vi "读取倍频程数据.vi"(8 "error in (no error)":errorcluster caption="错误输入（无错误）", 10 "写入缓冲区":string, 11 "设备选择":refnum<visa-resource-name>) -> (0 "error out":errorcluster caption="错误输出", 1 "read OCT":string, 2 "read SLM":string, 3 "通道编号输出":u32)   [LabVIEW 2020, in "bas_meas.lvlib"]
uses:
  bas_meas.lvlib
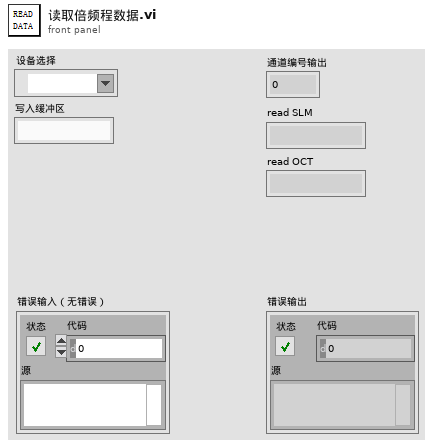
[diagram p1: front panel]
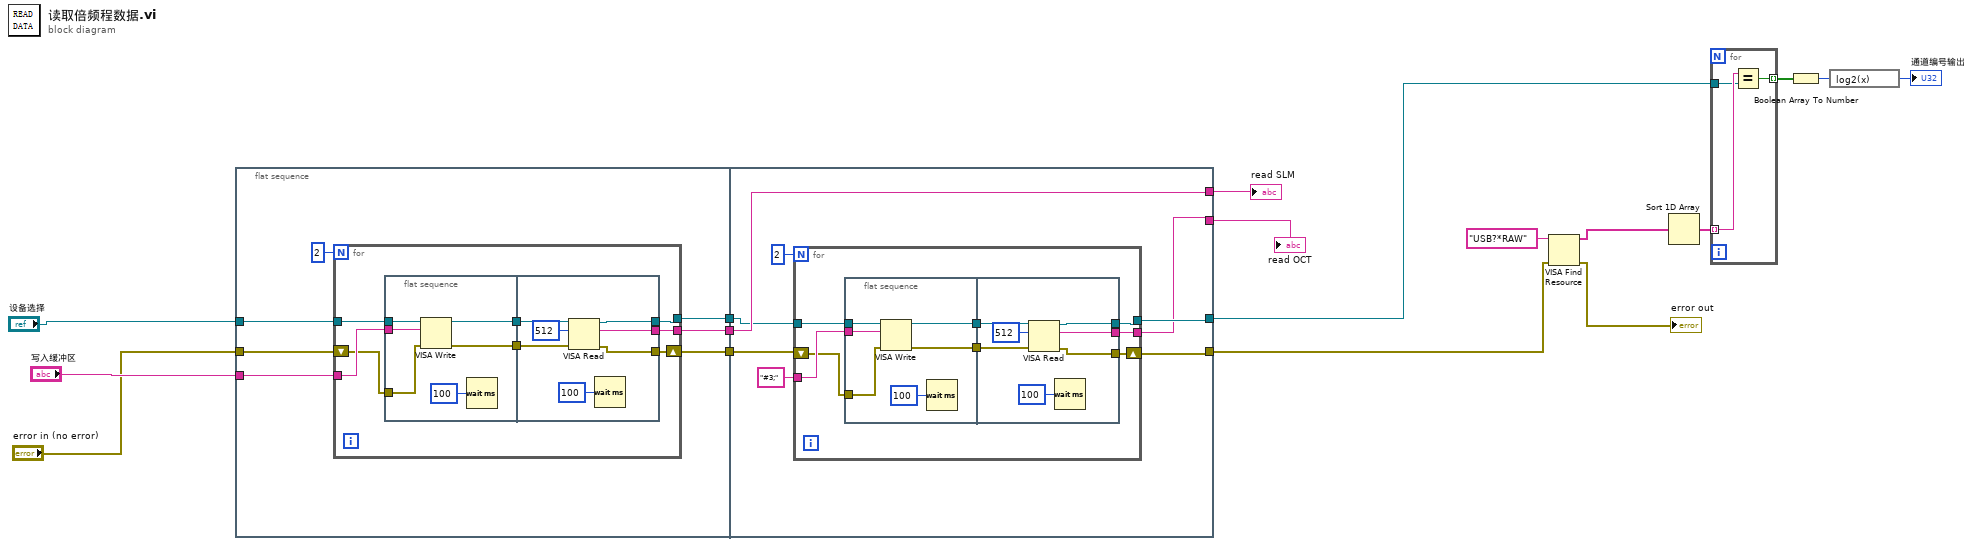
[diagram p0: block diagram]
diagram:
  n1 = flat-sequence {
    tunnel: "设备选择" -> [w24]
    tunnel: "写入缓冲区" -> [w23]
    tunnel: "error in (no error)" -> [w20]
    tunnel: [w22] -> w5
    tunnel: [w19] -> w4
    tunnel: [w18] -> w3
    tunnel: [w48] -> w6
    tunnel: [w46] -> w9
    tunnel: w5 -> [w52]
    tunnel: w4 -> [w50]
    tunnel: w3 -> [w51]
    tunnel: [w52] -> w2
    tunnel: [w47] -> w1
    frame #0 {
      n2 = for {
        N: 2 -> [_]
        tunnel: w24 -> [w30]
        tunnel: w23 -> [w29]
        tunnel: [w28] -> w22
        shift-right: [w27] -> w19
        shift-left: w20 -> [w26]
        tunnel: [w25] -> w18
        n3 = flat-sequence {
          tunnel: w30 -> [w38]
          tunnel: w29 -> [w37]
          tunnel: [w36] -> w32
          tunnel: [w35] -> w31
          tunnel: w26 -> [w33]
          tunnel: w32 -> [w45]
          tunnel: w31 -> [w44]
          tunnel: [w43] -> w28
          tunnel: [w40] -> w27
          tunnel: [w39] -> w25
          frame #0 {
            n4 = VISA Write(VISA resource name=w38, write buffer=w37, error in (no error)=w33) -> (VISA resource name out=w36:refnum<visa-resource-name>, error out=w35:errorcluster)  [unwired: 1 out]
            n5 = Wait (ms)(milliseconds to wait=u32 100 ("等待时间（毫秒）")) -> ()  [unwired: 1 out]
          }
          frame #1 {
            n6 = VISA Read(VISA resource name=w45, byte count=u32 512 ("字节总数"), error in (no error)=w44) -> (VISA resource name out=w39:refnum<visa-resource-name>, read buffer=w43:string, error out=w40:errorcluster)  [unwired: 1 out]
            n7 = Wait (ms)(milliseconds to wait=u32 100 ("等待时间（毫秒）")) -> ()  [unwired: 1 out]
          }
        }
      }
    }
    frame #1 {
      n8 = for {
        N: 2 -> [_]
        tunnel: w51 -> [w59]
        tunnel: "#3;" ("写入缓冲区") -> [w58]
        tunnel: [w57] -> w47
        shift-right: [w56] -> w46
        shift-left: w50 -> [w55]
        tunnel: [w54] -> w48
        n9 = flat-sequence {
          tunnel: w59 -> [w67]
          tunnel: w58 -> [w66]
          tunnel: [w65] -> w61
          tunnel: [w64] -> w60
          tunnel: w55 -> [w62]
          tunnel: w61 -> [w74]
          tunnel: w60 -> [w73]
          tunnel: [w72] -> w57
          tunnel: [w69] -> w56
          tunnel: [w68] -> w54
          frame #0 {
            n10 = VISA Write(VISA resource name=w67, write buffer=w66, error in (no error)=w62) -> (VISA resource name out=w65:refnum<visa-resource-name>, error out=w64:errorcluster)  [unwired: 1 out]
            n11 = Wait (ms)(milliseconds to wait=u32 100 ("等待时间（毫秒）")) -> ()  [unwired: 1 out]
          }
          frame #1 {
            n12 = VISA Read(VISA resource name=w74, byte count=u32 512 ("字节总数"), error in (no error)=w73) -> (VISA resource name out=w68:refnum<visa-resource-name>, read buffer=w72:string, error out=w69:errorcluster)  [unwired: 1 out]
            n13 = Wait (ms)(milliseconds to wait=u32 100 ("等待时间（毫秒）")) -> ()  [unwired: 1 out]
          }
        }
      }
    }
  }
  n14 = VISA Find Resource(8:w9, 11:"USB?*RAW" ("表达式(\"?*\")")) -> (0:→"error out":errorcluster, 3:w15:string[])  [unwired: 1 in, 1 out]
  n15 = Sort 1D Array(array=w15) -> (sorted array=w14:string[])
  n16 = for {
    tunnel: w14 -> [w77] mode=indexing
    tunnel: [w76] -> w13 mode=indexing
    tunnel: w6 -> [w75]
    n17 = Equal?(x=w77, y=w75) -> (x = y?=w76:bool)
  }
  n18 = Boolean Array To Number(Boolean array=w13) -> (number=w12:u32)
  n19 = expression code="log2(x)"(w12) -> (→"通道编号输出":u32)
  "read SLM" <- w2
  "read OCT" <- w1
